vi "List File Path Array.vi"(8 "error in":errorcluster, 11 "Files folder":path) -> (0 "error out":errorcluster, 3 "File Array out":string[](array[string]))   [LabVIEW 2018]
uses:
  <vilib>/Utility/error.llb/Error Cluster From Error Code.vi
  <vilib>/ErrorRing/Error Ring.xnode
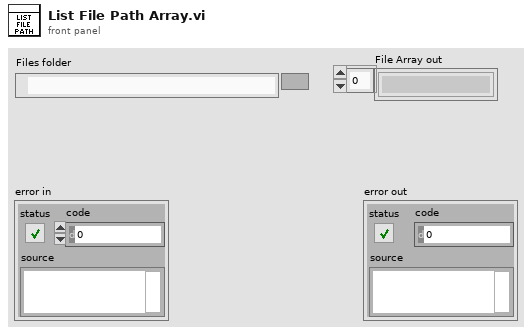
[diagram p1: front panel]
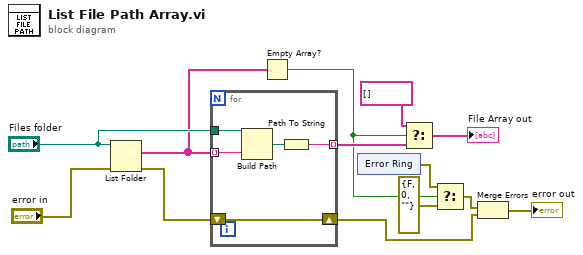
[diagram p0: block diagram]
diagram:
  n1 = List Folder(path="Files folder", error in="error in") -> (filenames=w10:string[], error out=w12:errorcluster)  [unwired: 2 in, 2 out]
  n2 = for {
    shift-right: [w16] -> w2
    shift-left: w12 -> [w16]
    tunnel: w10 -> [w17] mode=indexing
    tunnel: "Files folder" -> [w18]
    tunnel: [w14] -> w8 mode=indexing
    n3 = Build Path(base path=w18, name or relative path=w17) -> (appended path=w15:path)
    n4 = Path To String(path=w15) -> (string=w14:string)
  }
  n5 = Empty Array?(array=w10) -> (empty?=w6:bool)
  n6 = xnode "Error Ring"() -> ("error out"=w5:errorcluster)
  n7 = Select(t=string[] [] ("File Array out"), s=w6, f=w8) -> (s? t:f=→"File Array out":string[])
  n8 = Select(t=w5, s=w6, f=errorcluster {"status"=FALSE, "code"=0, "source"=""}) -> (s? t:f=w3:errorcluster)
  n9 = Merge Errors(w3, w2) -> (→"error out":errorcluster)
